vi "SaveParamImages.vi"(0 "Directory Parh":path, 1 "Data Formats":T2(ring), 2 "file name":string, 3 "Range Params":T4 {"int min" format="%.2f"; "int max" format="%.2f"; "slope min" format="%.2f"; "slope max" format="%.2f"; "mb min" format="%.2f"; "mb max" format="%.2f"}, 5 "slope":dbl[][](array[numeric]) format="%.2f", 7 "Header In":T1={"header info"={"Header"="", "Head length"=0}, "A/D info"={"# rf points per line"=0, "# lines per scan"=0, "sample rate MHz"=0, "# A/D bits"=0, "# bytes per A/D"=0, "TGC Flag"=0, "A/D Type"=""}, "Tranducer Info"={"bandwidth"=0.0, "center freq"=0.0, "start freq"=0.0, "ID"=0}, "Scan Info"={"delay"=0.0, "pivot distance"=0.0, "sector scan angle"=0.0, "operator"="", "Scan Mode"="", "location"=""}, "Time/Date Info"={"date"="", "time"=""}, "RF Info"={"RF file name"="", "RF file att"="", "RF cal file name"="", "RF cal file att"=""}, "Patient Info"={"ID"="", "extended ID"="", "age"=0, "sex"="", "previously\nscanned"="", "PSA"=0.0, "LOS"=1, "Ethnicty 2"=3, "Race"=3}, "Tissue Type"={"organ"=0, "disease type"=0, "disease location"=0, "IQ_pts"=0, "RcvBuffer"=0, "RcvFrame"=0, "IQBuff"=0, "IQFrame"=0, "IQPage"=0}, "Votage scaling"={"Digitizer (dB)"=0.0, "Gain (dB)"=0.0, "Atten (dB)"=0.0}, "Comment"="", "Misc Info"={"avg num"=0, "c speed"=0, "Div By or SF zones"=0, "XMIT CHS"=0, "RCV CHS"=0, "Xmit angle"=0.0}, "Therapy Parameters"={"Theraputic Freq (MHz)"=0.1, "Time on (s)"=1.0, "Therapy amplitude (mV)"=50.0, "Lines Before"=20, "Lines After"=80}, "Scan Settings"={"Energy (uJ or V)"=0, "Damp (Ohm) or Fc"=0, "HP Filt (KHz)"=0, "LP Filt (MHz)"=0, "Gain (db)"=0, "prf (kHz)"=0.0, "Distance between\nscan lines (um)"=0, "Distance between\nscan planes (um)"=0, "Scan line gap (um)"=0.0, "Scan plane gap (um)"=0.0}, "Compression Parameters"={"F1 (MHz)"=0.0, "F2 (MHz)"=0.0, "% taper"=0.0, "duration"=0.0}, "Patient Info Xtra"={"First Name"="", "Last Name"="", "Notes"=""}, "ROI Box"=[]} {"Compression Parameters"."% taper" min=50 max=1000 format="%.2f"; "Compression Parameters"."F2 (MHz)" format="%.3f"; "Compression Parameters"."F1 (MHz)" format="%.3f"; "Scan Settings"."prf (kHz)" format="%.2f"; "Therapy Parameters"."Therapy amplitude (mV)" min=50 max=1000 format="%.2f"; "Therapy Parameters"."Time on (s)" format="%.3f"; "Therapy Parameters"."Theraputic Freq (MHz)" format="%.3f"; "Patient Info"."Race" items=["Am Ind or Alaska", "Asian", "Hawaiian, Pac Isl", "Black or Afr Amer", "White", "more than one race", "unknown"]; "Patient Info"."Ethnicty 2" items=["Hispanic", "Non-Hispanic", "unknown"]; "Patient Info"."LOS" items=["1", "2", "3", "4", "5"]; "Patient Info"."PSA" format="%.1f"; "Scan Info"."delay" format="%.2f"; "Scan Info"."pivot distance" format="%.2f"; "Scan Info"."sector scan angle" format="%.2f"; "Tranducer Info"."bandwidth" format="%.2f"; "Tranducer Info"."center freq" format="%.2f"; "Tranducer Info"."start freq" format="%.2f"}, 9 "intercept":dbl[][](array[numeric]) format="%.2f", 11 "midband fit":dbl[][](array[numeric]) format="%.2f", 13 "Final Image Size":T3={"x"=346, "y"=240, "Trim image sides?"=FALSE, "start trim"=45, "end trim line"=256}) -> ()   [LabVIEW 2022 SP3]
uses:
  ViewData/-ReadEye/Header.ctl
  <vilib>/Utility/file.llb/Write Delimited Spreadsheet (DBL).vi
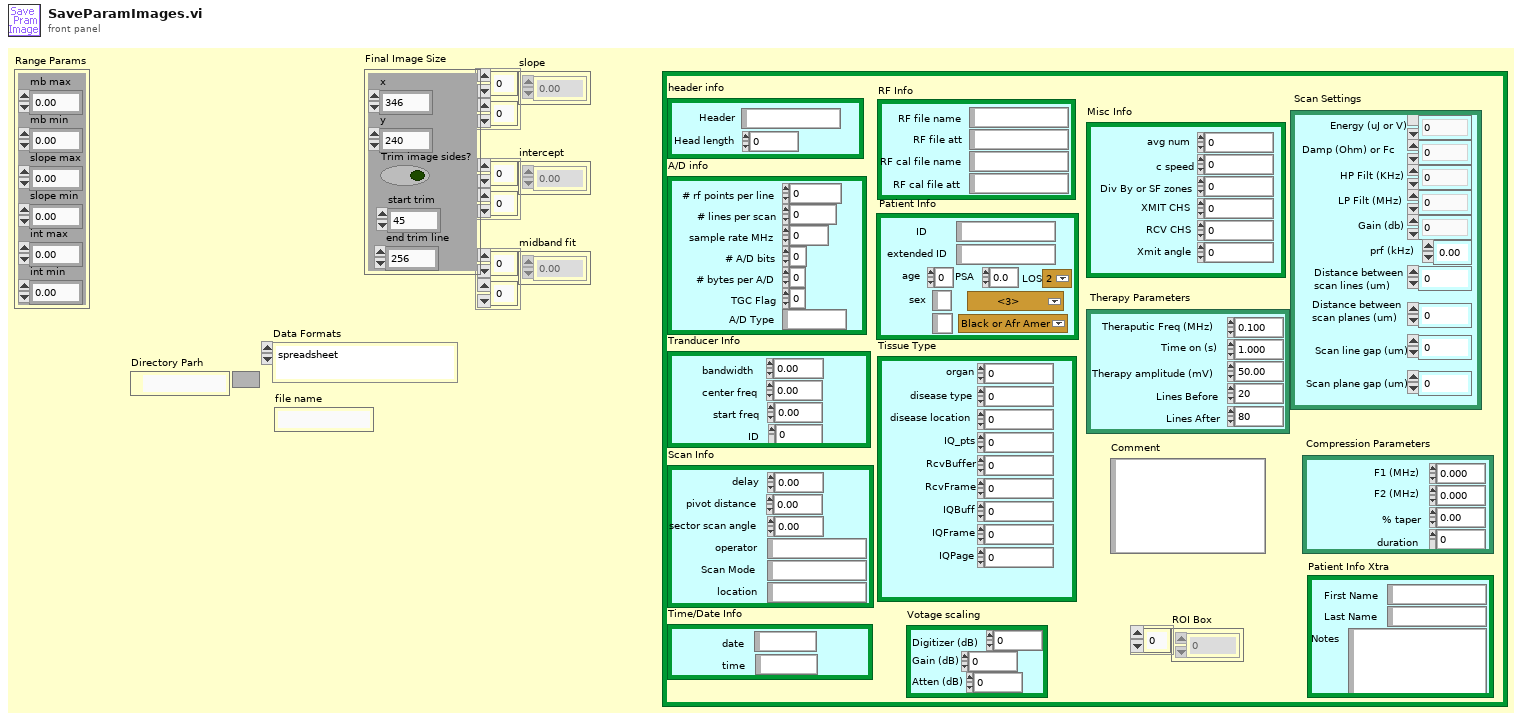
[diagram p1: front panel]
types:
  T1 = typedef "Header.ctl" = cluster{"header info":cluster{"Header":string, "Head length":i16}, "A/D info":cluster{"# rf points per line":u16, "# lines per scan":u16, "sample rate MHz":u16, "# A/D bits":i16, "# bytes per A/D":u16, "TGC Flag":u16, "A/D Type":string}, "Tranducer Info":cluster{"bandwidth":sgl, "center freq":sgl, "start freq":sgl, "ID":i32}, "Scan Info":cluster{"delay":sgl, "pivot distance":sgl, "sector scan angle":sgl, "operator":string, "Scan Mode":string, "location":string}, "Time/Date Info":cluster{"date":string, "time":string}, "RF Info":cluster{"RF file name":string, "RF file att":string, "RF cal file name":string, "RF cal file att":string}, "Patient Info":cluster{"ID":string, "extended ID":string, "age":u16, "sex":string, "previously\nscanned":string, "PSA":sgl, "LOS":u8, "Ethnicty 2":u8, "Race":u8}, "Tissue Type":cluster{"organ":i16, "disease type":i16, "disease location":i16, "IQ_pts":u16, "RcvBuffer":u8, "RcvFrame":u16, "IQBuff":u8, "IQFrame":u16, "IQPage":u8}, "Votage scaling":cluster{"Digitizer (dB)":sgl, "Gain (dB)":sgl, "Atten (dB)":sgl}, "Comment":string, "Misc Info":cluster{"avg num":u16, "c speed":i16, "Div By or SF zones":i16, "XMIT CHS":u8, "RCV CHS":u8, "Xmit angle":sgl}, "Therapy Parameters":cluster{"Theraputic Freq (MHz)":sgl, "Time on (s)":sgl, "Therapy amplitude (mV)":sgl, "Lines Before":u16, "Lines After":u16}, "Scan Settings":cluster{"Energy (uJ or V)":u8, "Damp (Ohm) or Fc":u8, "HP Filt (KHz)":u8, "LP Filt (MHz)":u8, "Gain (db)":u8, "prf (kHz)":sgl, "Distance between\nscan lines (um)":u16, "Distance between\nscan planes (um)":u16, "Scan line gap (um)":sgl, "Scan plane gap (um)":sgl}, "Compression Parameters":cluster{"F1 (MHz)":sgl, "F2 (MHz)":sgl, "% taper":sgl, "duration":sgl}, "Patient Info Xtra":cluster{"First Name":string, "Last Name":string, "Notes":string}, "ROI Box":u16[]}
  T2 = enum16{"spreadsheet", "8 bit byte file", "sector byte file", "8 bit BMP file", "sector 8 bit BMP file"}
  T3 = cluster{"x":i32, "y":i32, "Trim image sides?":bool, "start trim":i32, "end trim line":i32}
  T4 = cluster{"mb max":dbl, "mb min":dbl, "slope max":dbl, "slope min":dbl, "int max":dbl, "int min":dbl}
  T5 = cluster{"# rf points per line":u16, "# lines per scan":u16, "sample rate MHz":u16, "# A/D bits":i16, "# bytes per A/D":u16, "TGC Flag":u16, "A/D Type":string}
  T6 = cluster{"delay":sgl, "pivot distance":sgl, "sector scan angle":sgl, "operator":string, "Scan Mode":string, "location":string}
  T7 = enum16{"open", "replace", "create", "open or create", "replace or create", "replace or create with confirmation"}
  T8 = typedef "imagedata.ctl" = cluster{"image type":i32, "image depth":i32, "image":u8[], "mask":u8[], "colors":u32[], "Rectangle":cluster{"left":i16, "top":i16, "right":i16, "bottom":i16}}
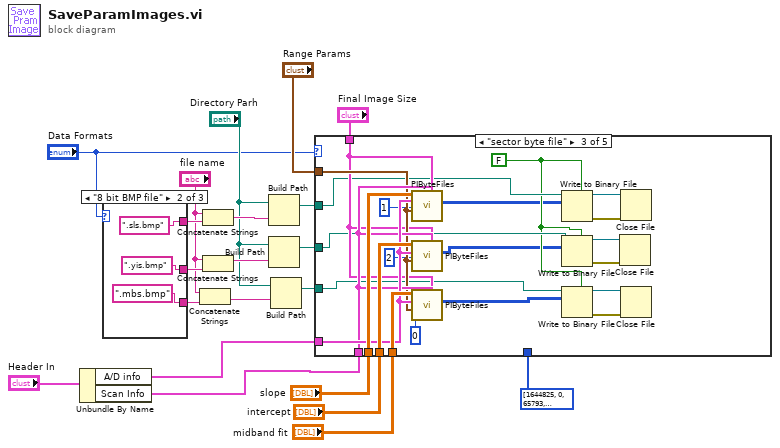
[diagram p0: block diagram]
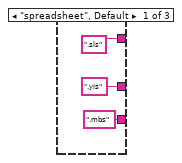
[diagram p2: hidden frame]
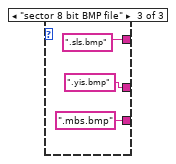
[diagram p3: hidden frame]
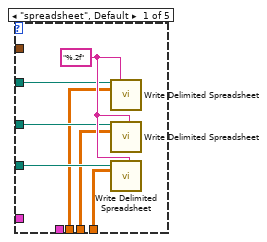
[diagram p4: hidden frame]
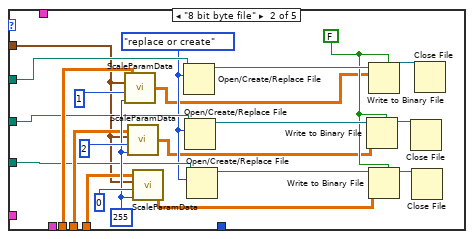
[diagram p5: hidden frame]
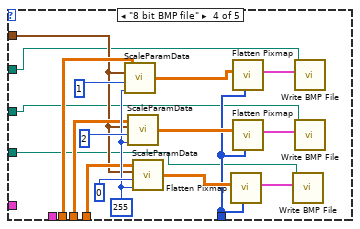
[diagram p6: hidden frame]
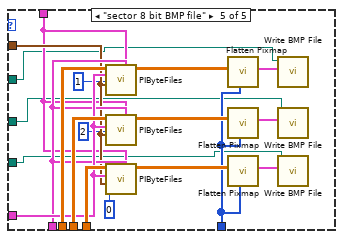
[diagram p7: hidden frame]
diagram:
  n1 = Unbundle By Name("Header In") -> ("A/D info"=w2:T5, "Scan Info"=w1:T6)
  n2 = case shown="\"8 bit BMP file\"" "Data Formats" {
    tunnel: [".mbs" ".mbs.bmp" ".mbs.bmp"] -> w14
    tunnel: [".yis" ".yis.bmp" ".yis.bmp"] -> w13
    tunnel: [".sls" ".sls.bmp" ".sls.bmp"] -> w12
    frame "spreadsheet", Default {
    }
    frame "8 bit BMP file" {
    }
    frame "sector 8 bit BMP file" {
    }
  }
  n3 = Concatenate Strings("file name", w14) -> (w17:string)
  n4 = Concatenate Strings("file name", w12) -> (w15:string)
  n5 = Concatenate Strings("file name", w13) -> (w16:string)
  n6 = Build Path(base path="Directory Parh", name or relative path=w15) -> (appended path=w11:path)
  n7 = Build Path(base path="Directory Parh", name or relative path=w16) -> (appended path=w10:path)
  n8 = Build Path(base path="Directory Parh", name or relative path=w17) -> (appended path=w9:path)
  n9 = case shown="\"sector byte file\"" "Data Formats" {
    tunnel: "slope" -> [w33 w50 w82 w96 w120]
    tunnel: "intercept" -> [w32 w49 w81 w95 w119]
    tunnel: "midband fit" -> [w31 w48 w80 w94 w118]
    tunnel: w2 -> [_ _ w79 _ w117]
    tunnel: w1 -> [_ _ w78 _ w116]
    tunnel: "Range Params" -> [_ w44 w77 w93 w115]
    tunnel: w11 -> [w36 w45 w72 w86 w103]
    tunnel: w10 -> [w35 w46 w71 w85 w101]
    tunnel: w9 -> [w34 w47 w70 w84 w102]
    tunnel: "Final Image Size" -> [_ _ w73 _ w111]
    tunnel: u32[] [1644825, 0, 65793, 131586, 197379, 263172, 328965, 394758, 460551, 526344, 592137, 657930, 723723, 789516, 855309, 921102, 986895, 1052688, 1118481, 1184274, 1250067, 1315860, 1381653, 1447446, 1513239, 1579032, 1644825, 1710618, 1776411, 1842204, 1907997, 1973790, 2039583, 2105376, 2171169, 2236962, 2302755, 2368548, 2434341, 2500134, 2565927, 2631720, 2697513, 2763306, 2829099, 2894892, 2960685, 3026478, 3092271, 3158064, 3223857, 3289650, 3355443, 3421236, 3487029, 3552822, 3618615, 3684408, 3750201, 3815994, 3881787, 3947580, 4013373, 4079166, 4144959, 4210752, 4276545, 4342338, 4408131, 4473924, 4539717, 4605510, 4671303, 4737096, 4802889, 4868682, 4934475, 5000268, 5066061, 5131854, 5197647, 5263440, 5329233, 5395026, 5460819, 5526612, 5592405, 5658198, 5723991, 5789784, 5855577, 5921370, 5987163, 6052956, 6118749, 6184542, 6250335, 6316128, 6381921, 6447714, 6513507, 6579300, 6645093, 6710886, 6776679, 6842472, 6908265, 6974058, 7039851, 7105644, 7171437, 7237230, 7303023, 7368816, 7434609, 7500402, 7566195, 7631988, 7697781, 7763574, 7829367, 7895160, 7960953, 8026746, 8092539, 8158332, 8224125, 8289918, 8355711, 8421504, 8487297, 8553090, 8618883, 8684676, 8750469, 8816262, 8882055, 8947848, 9013641, 9079434, 9145227, 9211020, 9276813, 9342606, 9408399, 9474192, 9539985, 9605778, 9671571, 9737364, 9803157, 9868950, 9934743, 10000536, 10066329, 10132122, 10197915, 10263708, 10329501, 10395294, 10461087, 10526880, 10592673, 10658466, 10724259, 10790052, 10855845, 10921638, 10987431, 11053224, 11119017, 11184810, 11250603, 11316396, 11382189, 11447982, 11513775, 11579568, 11645361, 11711154, 11776947, 11842740, 11908533, 11974326, 12040119, 12105912, 12171705, 12237498, 12303291, 12369084, 12434877, 12500670, 12566463, 12632256, 12698049, 12763842, 12829635, 12895428, 12961221, 13027014, 13092807, 13158600, 13224393, 13290186, 13355979, 13421772, 13487565, 13553358, 13619151, 13684944, 13750737, 13816530, 13882323, 13948116, 14013909, 14079702, 14145495, 14211288, 14277081, 14342874, 14408667, 14474460, 14540253, 14606046, 14671839, 14737632, 14803425, 14869218, 14935011, 15000804, 15066597, 15132390, 15198183, 15263976, 15329769, 15395562, 15461355, 15527148, 15592941, 15658734, 15724527, 15790320, 15856113, 15921906, 15987699, 16053492, 16119285, 16185078, 16250871, 16316664, 16382457, 16448250, 16514043, 16579836, 16645629, 16711680] ("Color Table") -> [_ _ _ w87 w104]
    frame "spreadsheet", Default {
      w37 = "%.2f"
      n10 = call-poly <vilib>:"Write Delimited Spreadsheet.vi"("file path (dialog if empty)"=w36, "format (%.3f)"=w37, "2D data"=w33) -> ()  [unwired: 11 in, 2 out]
      n11 = call-poly <vilib>:"Write Delimited Spreadsheet.vi"("file path (dialog if empty)"=w35, "format (%.3f)"=w37, "2D data"=w32) -> ()  [unwired: 11 in, 2 out]
      n12 = call-poly <vilib>:"Write Delimited Spreadsheet.vi"("file path (dialog if empty)"=w34, "format (%.3f)"=w37, "2D data"=w31) -> ()  [unwired: 11 in, 2 out]
    }
    frame "8 bit byte file" {
      w42 = T7."replace or create" ("operation (0:open)")
      w41 = FALSE ("prepend array or string size? (T)")
      w54 = 255
      n13 = call "ScaleParamData.vi"("max scale value"=w54, "parameter"=1, "Range Params"=w44, "raw image data in"=w50) -> ("scaled output"=w40:dbl[][])
      n14 = call "ScaleParamData.vi"("max scale value"=w54, "parameter"=2, "Range Params"=w44, "raw image data in"=w49) -> ("scaled output"=w39:dbl[][])
      n15 = call "ScaleParamData.vi"("max scale value"=w54, "parameter"=0, "Range Params"=w44, "raw image data in"=w48) -> ("scaled output"=w38:dbl[][])
      n16 = Open/Create/Replace File(file path (use dialog)=w45, operation (0:open)=w42) -> (refnum out=w43:refnum<file>)  [unwired: 1 in, 5 out]
      n17 = Open/Create/Replace File(file path (use dialog)=w46, operation (0:open)=w42) -> (refnum out=w56:refnum<file>)  [unwired: 1 in, 5 out]
      n18 = Open/Create/Replace File(file path (use dialog)=w47, operation (0:open)=w42) -> (refnum out=w55:refnum<file>)  [unwired: 1 in, 5 out]
      n19 = Write to Binary File(file (use dialog)=w56, data=w39, 5:w41) -> (refnum out=w53:refnum<file>)  [unwired: 1 in, 4 out]
      n20 = Write to Binary File(file (use dialog)=w43, data=w40, 5:w41) -> (refnum out=w52:refnum<file>)  [unwired: 1 in, 4 out]
      n21 = Write to Binary File(file (use dialog)=w55, data=w38, 5:w41) -> (refnum out=w51:refnum<file>)  [unwired: 1 in, 4 out]
      n22 = Close File(refnum=w53) -> ()  [unwired: 1 in, 2 out]
      n23 = Close File(refnum=w51) -> ()  [unwired: 1 in, 2 out]
      n24 = Close File(refnum=w52) -> ()  [unwired: 1 in, 2 out]
    }
    frame "sector byte file" {
      w63 = FALSE ("prepend array or string size? (T)")
      n25 = call "PIByteFiles.vi"("Final Sector Image Size"=w73, "Scan Info"=w78, "Data Type"=1, "Range Params"=w77, "A/D info"=w79, "raw image data in"=w82) -> ("Scaled Image Data"=w62:u8[][])  [unwired: 3 in, 2 out]
      n26 = call "PIByteFiles.vi"("Final Sector Image Size"=w73, "Scan Info"=w78, "Data Type"=2, "Range Params"=w77, "A/D info"=w79, "raw image data in"=w81) -> ("Scaled Image Data"=w61:u8[][])  [unwired: 3 in, 2 out]
      n27 = call "PIByteFiles.vi"("Final Sector Image Size"=w73, "Scan Info"=w78, "Data Type"=0, "Range Params"=w77, "A/D info"=w79, "raw image data in"=w80) -> ("Scaled Image Data"=w60:u8[][])  [unwired: 3 in, 2 out]
      n28 = Write to Binary File(file (use dialog)=w72, data=w62, 5:w63) -> (refnum out=w68:refnum<file>, error out=w69:errorcluster)  [unwired: 1 in, 3 out]
      n29 = Write to Binary File(file (use dialog)=w71, data=w61, 5:w63) -> (refnum out=w65:refnum<file>, error out=w64:errorcluster)  [unwired: 1 in, 3 out]
      n30 = Write to Binary File(file (use dialog)=w70, data=w60, 5:w63) -> (refnum out=w67:refnum<file>, error out=w66:errorcluster)  [unwired: 1 in, 3 out]
      n31 = Close File(refnum=w65, error in=w64) -> ()  [unwired: 2 out]
      n32 = Close File(refnum=w68, error in=w69) -> ()  [unwired: 2 out]
      n33 = Close File(refnum=w67, error in=w66) -> ()  [unwired: 2 out]
    }
    frame "8 bit BMP file" {
      w97 = 255
      n34 = call "ScaleParamData.vi"("max scale value"=w97, "parameter"=1, "Range Params"=w93, "raw image data in"=w96) -> ("scaled output"=w83:dbl[][])
      n35 = call "ScaleParamData.vi"("max scale value"=w97, "parameter"=2, "Range Params"=w93, "raw image data in"=w95) -> ("scaled output"=w88:dbl[][])
      n36 = call "ScaleParamData.vi"("max scale value"=w97, "parameter"=0, "Range Params"=w93, "raw image data in"=w94) -> ("scaled output"=w92:dbl[][])
      n37 = call <vilib>:"Flatten Pixmap.vi"("colors"=w87, "8-bit pixmap"=w92) -> ("image data"=w89:T8)  [unwired: 4 in, 5 out]
      n38 = call <vilib>:"Flatten Pixmap.vi"("colors"=w87, "8-bit pixmap"=w83) -> ("image data"=w91:T8)  [unwired: 4 in, 5 out]
      n39 = call <vilib>:"Flatten Pixmap.vi"("colors"=w87, "8-bit pixmap"=w88) -> ("image data"=w90:T8)  [unwired: 4 in, 5 out]
      n40 = call <vilib>:"Write BMP File.vi"("image data"=w89, "path to BMP file"=w84) -> ()  [unwired: 2 in, 8 out]
      n41 = call <vilib>:"Write BMP File.vi"("image data"=w91, "path to BMP file"=w86) -> ()  [unwired: 2 in, 8 out]
      n42 = call <vilib>:"Write BMP File.vi"("image data"=w90, "path to BMP file"=w85) -> ()  [unwired: 2 in, 8 out]
    }
    frame "sector 8 bit BMP file" {
      n43 = call "PIByteFiles.vi"("Final Sector Image Size"=w111, "Scan Info"=w116, "Data Type"=1, "Range Params"=w115, "A/D info"=w117, "raw image data in"=w120) -> ("raw sector out"=w106:dbl[][])  [unwired: 3 in, 2 out]
      n44 = call "PIByteFiles.vi"("Final Sector Image Size"=w111, "Scan Info"=w116, "Data Type"=2, "Range Params"=w115, "A/D info"=w117, "raw image data in"=w119) -> ("raw sector out"=w107:dbl[][])  [unwired: 3 in, 2 out]
      n45 = call "PIByteFiles.vi"("Final Sector Image Size"=w111, "Scan Info"=w116, "Data Type"=0, "Range Params"=w115, "A/D info"=w117, "raw image data in"=w118) -> ("raw sector out"=w105:dbl[][])  [unwired: 3 in, 2 out]
      n46 = call <vilib>:"Flatten Pixmap.vi"("colors"=w104, "8-bit pixmap"=w106) -> ("image data"=w110:T8)  [unwired: 4 in, 5 out]
      n47 = call <vilib>:"Flatten Pixmap.vi"("colors"=w104, "8-bit pixmap"=w107) -> ("image data"=w109:T8)  [unwired: 4 in, 5 out]
      n48 = call <vilib>:"Flatten Pixmap.vi"("colors"=w104, "8-bit pixmap"=w105) -> ("image data"=w108:T8)  [unwired: 4 in, 5 out]
      n49 = call <vilib>:"Write BMP File.vi"("image data"=w110, "path to BMP file"=w103) -> ()  [unwired: 2 in, 8 out]
      n50 = call <vilib>:"Write BMP File.vi"("image data"=w109, "path to BMP file"=w101) -> ()  [unwired: 2 in, 8 out]
      n51 = call <vilib>:"Write BMP File.vi"("image data"=w108, "path to BMP file"=w102) -> ()  [unwired: 2 in, 8 out]
    }
  }
